vi "Get MenuClass.vi"(11 "listbox in":refnum<class "listbox.lvclass">) -> (2 "MenuClass":variant, 3 "listbox out":refnum<class "listbox.lvclass">)   [LabVIEW 2016, in "listbox.lvclass"]
uses:
  listbox.lvclass
  listbox.lvclass/listbox.ctl
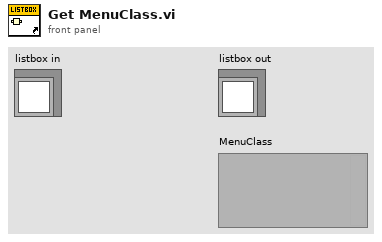
[diagram p1: front panel]
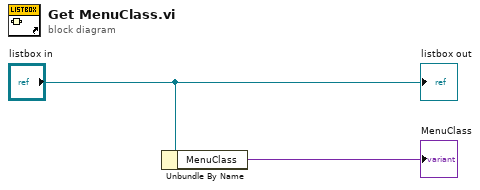
[diagram p0: block diagram]
diagram:
  n1 = Unbundle By Name("listbox in") -> ("MenuClass"=→"MenuClass":variant)
  "listbox out" <- "listbox in"
